vi "Deviated_Result_API.vi"(0 "Device DVR In":refnum<data-value>, 11 "Error in":errorcluster) -> (4 "Device DVR Out":refnum<data-value>, 15 "Error Out":errorcluster)   [LabVIEW 2020, in "Device.lvclass"]
uses:
  Device.lvclass
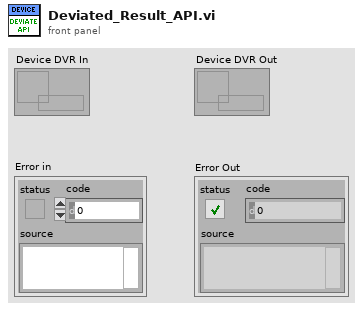
[diagram p1: front panel]
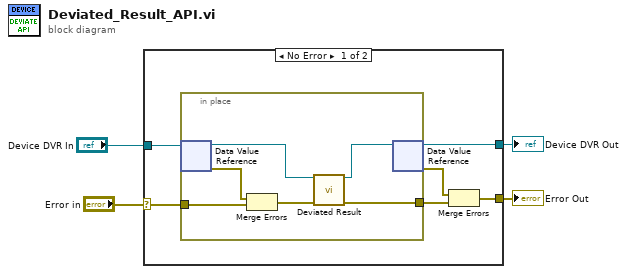
[diagram p0: block diagram]
diagram:
  n1 = case shown="No Error" "Error in" {
    selector: "Error in" -> [w10 w17]
    tunnel: "Device DVR In" -> [w9 w18]
    tunnel: [w6 w18] -> w2
    tunnel: [w5 w17] -> w1
    frame No Error {
      n2 = in-place {
        in-place-border: w10 -> [w16]
        in-place-border: [w11] -> w8
        n3 = in-place-dvr #1(w9) -> (w13:refnum<class "Device.lvclass">, w15:errorcluster)
        n4 = Merge Errors(w15, w16) -> (w14:errorcluster)
        n5 = call "Deviated Result.vi"("Device in"=w13, "Error in"=w14) -> ("Device out"=w12:refnum<class "Device.lvclass">, "Error out"=w11:errorcluster)  [unwired: 12 in]
        n6 = in-place-dvr #1(w12) -> (w6:refnum<data-value>, w7:errorcluster)
      }
      n7 = Merge Errors(w7, w8) -> (w5:errorcluster)
    }
    frame Error {
    }
  }
  "Device DVR Out" <- w2
  "Error Out" <- w1
